vi "Do.vi"(8 "error in (no error)":errorcluster, 10 "Actor in":refnum<class "Actor.lvclass">, 11 "Login Failure Msg":refnum<class "Login Failure Msg.lvclass">) -> (0 "error out":errorcluster, 2 "Actor out":refnum<class "Actor.lvclass">)   [LabVIEW 2017, in "Login View.lvlib" / "Login Failure Msg.lvclass"]
doc: "This VI delivers the message to the actor by calling the appropriate method(s) on the actor."
uses:
  <vilib>/gpm_packages/@cs/User Manager App/Login View/Login View Messages/Login Failure Msg/Login Failure Msg.lvclass
  <vilib>/ActorFramework/Actor/Actor.lvclass
  <vilib>/gpm_packages/@cs/User Manager App/Login View/Login View/Login View.lvclass
  C:/Program Files/National Instruments/LabVIEW 2017/vi.lib/ActorFramework/Actor/Actor.lvclass
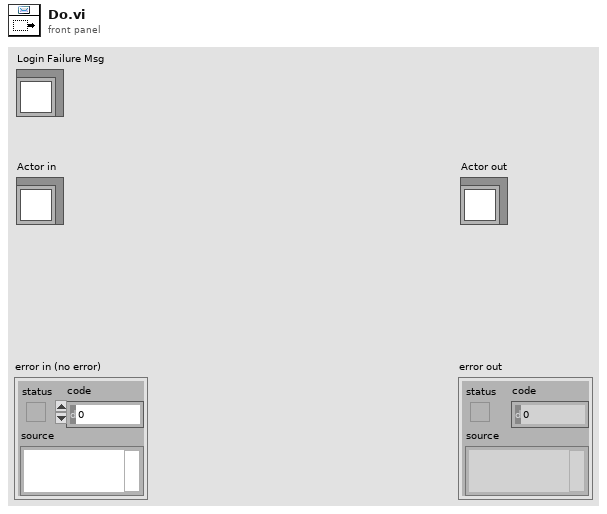
[diagram p1: front panel]
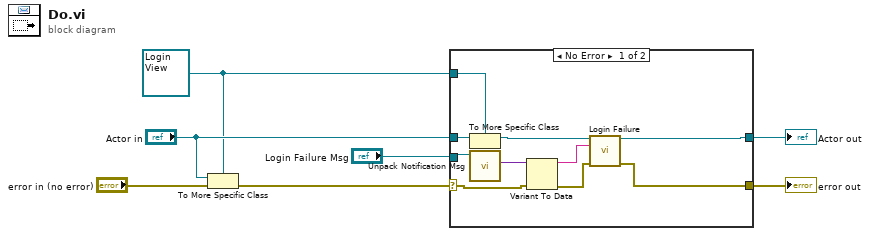
[diagram p0: block diagram]
diagram:
  w2 = refnum<class "Login View.lvclass"> refnum ("Actor in")
  n1 = To More Specific Class(target class=w2, reference="Actor in", error in="error in (no error)") -> (error out=w6:errorcluster)  [unwired: 1 out]
  n2 = case shown="No Error" w6 {
    selector: w6 -> [w9 w19]
    tunnel: [w17 w19] -> w5
    tunnel: [w16 w18] -> w4
    tunnel: "Actor in" -> [w15 w18]
    tunnel: w2 -> [w14 _]
    tunnel: "Login Failure Msg" -> [w12 _]
    frame No Error {
      n3 = To More Specific Class(target class=w14, reference=w15) -> (specific class reference=w13:refnum<class "Login View.lvclass">)  [unwired: 1 in, 1 out]
      n4 = call-dynamic "Unpack Notification Msg.vi"("Notification Msg"=w12) -> ("Value"=w11:variant)  [unwired: 8 in, 2 out]
      n5 = Variant To Data(error in=w9, Variant=w11) -> (data=w10:string, error out=w8:errorcluster)  [unwired: 1 in]
      n6 = call <vilib>:"Login Failure.vi"("Login View in"=w13, "Login Message"=w10, "error in (no error)"=w8) -> ("Login View out"=w16:refnum<class "Login View.lvclass">, "error out"=w17:errorcluster)  [unwired: 11 in]
    }
    frame Error {
      # "If type check fails, pass the original object out again."
    }
  }
  "error out" <- w5
  "Actor out" <- w4
